vi "Contains True.vi"(1 "R Channel BL":bool[](array[boolean])) -> (0 "Boolean":bool)   [LabVIEW 2019]
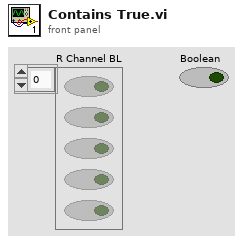
[diagram p1: front panel]
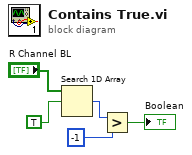
[diagram p0: block diagram]
diagram:
  n1 = Search 1D Array(1D array="R Channel BL", element=TRUE) -> (index of element=w3:i32)  [unwired: 1 in]
  n2 = Greater?(x=w3, y=-1) -> (0:→"Boolean":bool)
